vi "Data Contents Refresh__DV.vi"(8 "error in":errorcluster, 9 "Wfm Name":string[](array[string]), 10 "Graph Refreshed":waveform(dbl)[](array[waveform])) -> (0 "error out":errorcluster, 1 "Compute Result":string[][](array[string]))   [LabVIEW 2012]
doc: "本部分根据时间间隔以及Y值个数来得到屏幕上的时间长度。\n根据读出的2DDBL来计算最大最小值，以及峰峰值。"
uses:
  <vilib>/Analysis/baseanly.llb/Mean (DBL).vi
  <vilib>/Analysis/NI_AALBase.lvlib
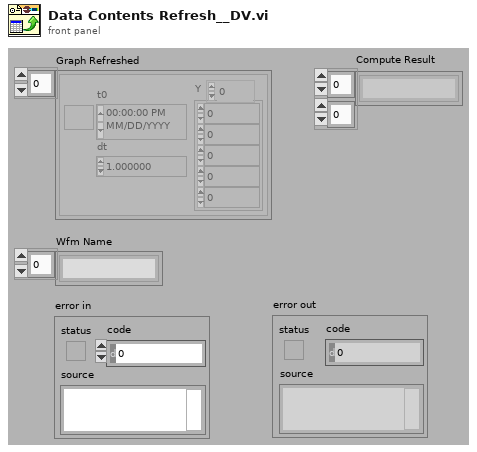
[diagram p1: front panel]
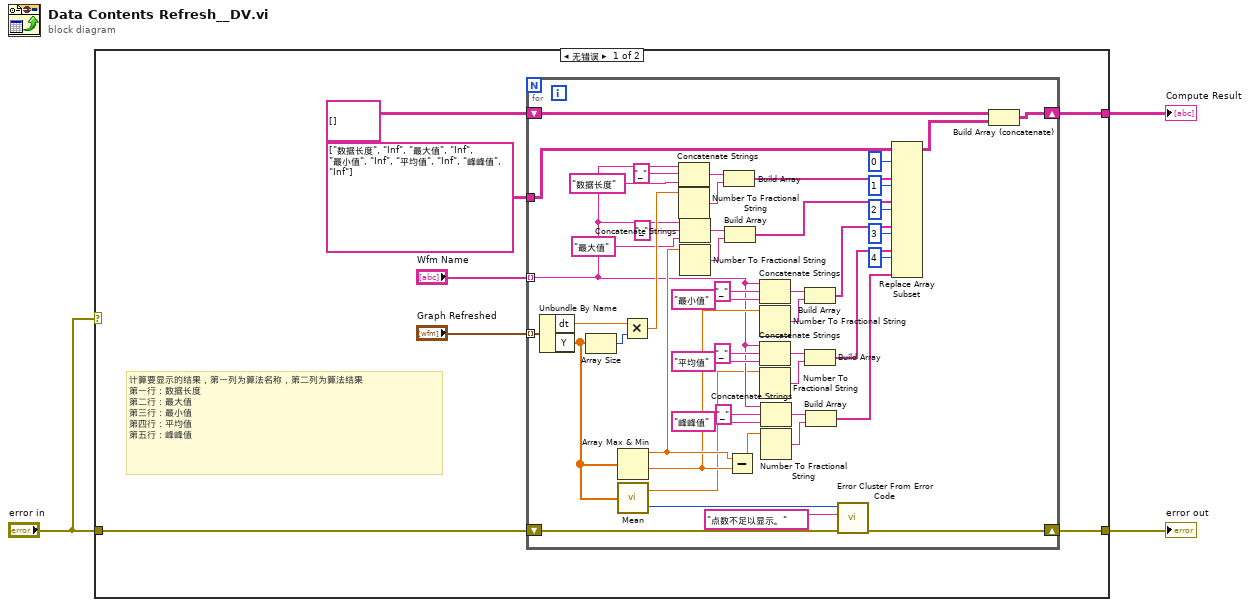
[diagram p0: block diagram]
diagram:
  n1 = case shown="无错误" "error in" {
    tunnel: "error in" -> [w9 w59]
    tunnel: [w7 w59] -> w3
    tunnel: [w4 _] -> w2
    frame No Error {
      # "计算要显示的结果，第一列为算法名称，第二列为算法结果\n第一行：数据长度\n第二行：最大值\n第三行：最小值\n第四行：平均值\n第五行：峰峰值"
      n2 = for {
        tunnel: "Graph Refreshed" -> [w58] mode=indexing
        tunnel: "Wfm Name" -> [w21] mode=indexing
        shift-right: [w52] -> w7
        shift-left: w9 -> [w53]
        tunnel: string[][] [["数据长度", "Inf"], ["最大值", "Inf"], ["最小值", "Inf"], ["平均值", "Inf"], ["峰峰值", "Inf"]] ("转置的数组") -> [w51]
        shift-right: [w11] -> w4
        shift-left: string[][] [] ("转置的数组") -> [w13]
        n3 = Unbundle By Name(w58) -> ("dt"=w57:dbl, "Y"=w39:dbl[])
        n4 = Array Size(array=w39) -> (size(s)=w56:i32)
        n5 = Array Max & Min(array=w39) -> (max value=w34:dbl, min value=w28:dbl)  [unwired: 2 out]
        n6 = call-poly <vilib>:"Mean.vi"("X"=w39) -> ("mean"=w19:dbl, "error"=w55:i32)
        n7 = Multiply(x=w57, y=w56) -> (x*y=w50:dbl)
        n8 = Concatenate Strings(w21, "_" ("字符串"), "数据长度") -> (w46:string)
        n9 = Number To Fractional String(number=w50) -> (F-format string=w45:string)  [unwired: 3 in]
        n10 = Concatenate Strings(w21, "_" ("字符串"), "最大值") -> (w37:string)
        n11 = Number To Fractional String(number=w34) -> (F-format string=w38:string)  [unwired: 3 in]
        n12 = Build Array(w46, w45) -> (w44:string[])
        n13 = Build Array(w37, w38) -> (w33:string[])
        n14 = Subtract(x=w34, y=w28) -> (x-y=w18:dbl)
        n15 = Concatenate Strings(w21, "_" ("字符串"), "最小值") -> (w30:string)
        n16 = Number To Fractional String(number=w28) -> (F-format string=w29:string)  [unwired: 3 in]
        n17 = Concatenate Strings(w21, "_" ("字符串"), "平均值") -> (w27:string)
        n18 = Number To Fractional String(number=w19) -> (F-format string=w17:string)  [unwired: 3 in]
        n19 = Concatenate Strings(w21, "_" ("字符串"), "峰峰值") -> (w22:string)
        n20 = Number To Fractional String(number=w18) -> (F-format string=w20:string)  [unwired: 3 in]
        n21 = Build Array(w30, w29) -> (w16:string[])
        n22 = Build Array(w27, w17) -> (w15:string[])
        n23 = Build Array(w22, w20) -> (w14:string[])
        n24 = call <vilib>:"Error Cluster From Error Code.vi"("error in (no error)"=w53, "error message (\"\")"="点数不足以显示。" ("error message (\"\")"), "error code (0)"=w55) -> ("error out"=w52:errorcluster)  [unwired: 6 in]
        n25 = Replace Array Subset(array=w51, new element #1=w44, index (row) #1=0 ("索引 (行)"), new element #2=w33, index (row) #2=1 ("索引 (行)"), new element #3=w16, index (row) #3=2 ("索引 (行)"), new element #4=w15, index (row) #4=3 ("索引 (行)"), new element #5=w14, index (row) #5=4 ("索引 (行)")) -> (w12:string[][])  [unwired: 5 in]
        n26 = Build Array (concatenate)(w13, w12) -> (w11:string[][])
      }
    }
    frame Error {
    }
  }
  "error out" <- w3
  "Compute Result" <- w2
